vi "Global_Drive_Encoders.vi"() -> ()   [LabVIEW 2017]
panel:
  in  "Drive encoders":T1
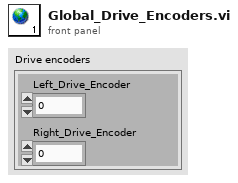
[diagram p1: front panel]
types:
  T1 = cluster{"Left_Drive_Encoder":i32, "Right_Drive_Encoder":i32}
diagram:
